vi "IO Module Testing.vi"() -> (0 "PIR":bool)   [LabVIEW 2015]
uses:
  <vilib>/rvi/interface/nirviOpenFPGA/nirviOpenFPGA.xnode
  <vilib>/rvi/interface/nirviMethod/nirviMethod.xnode
  <vilib>/FPGAPlugInAG/Dynamic/niLvFpga_Run_Dynamic.vi
  <vilib>/rvi/interface/nirviCloseFPGA/nirviCloseFPGA.xnode
  <vilib>/FPGAPlugInAG/Dynamic/niLvFpga_Close_Dynamic.vi
  FPGA Bitfiles/PDMSMain_FPGATarget-Wi-Fi_Express2_Jo8xc+hAvHc.lvbitx
  FPGA/Express.vi
  <vilib>/FPGAPlugInAG/myRIO-1900/niLvFpga_Open_myRIO-1900.vi
  <vilib>/rvi/interface/common/dynamic/niFpgaDynamicAddResources.vi
panel:
  out "Ultrasuond":cluster{"US BK":i16, "US FR":i16, "US FL":i16}
  out "Accelerometer":cluster{"Z":i16, "Y":i16, "X":i16}
  out "Button":bool
  out "Error Out":errorcluster
  in  "Error In":errorcluster
  in  "Stop Button":bool
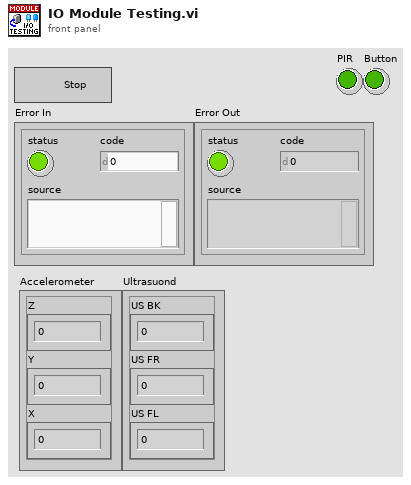
[diagram p1: front panel]
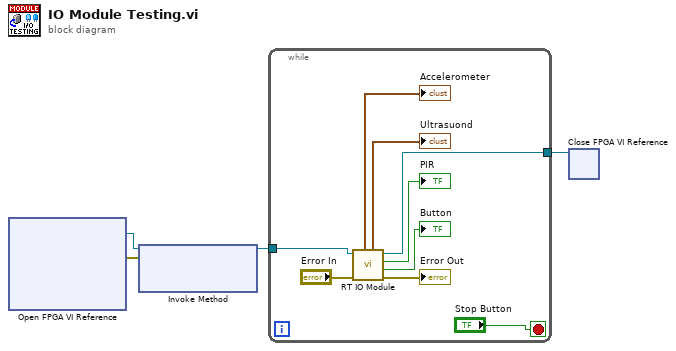
[diagram p0: block diagram]
diagram:
  n1 = xnode "Open FPGA VI Reference"() -> ("FPGA VI Reference Out"=w4:refnum<k20>, "error out"=w3:errorcluster)  [unwired: 2 in]
  n2 = xnode "Invoke Method"("FPGA VI Reference In"=w4, "error in"=w3) -> ("FPGA VI Reference Out"=w2:refnum<k20>)  [unwired: 1 in, 1 out]
  n3 = while {
    tunnel: w2 -> [w6]
    tunnel: [w5] -> w1
    stop <- "Stop Button" stop-if-true
    n4 = call "RT IO Module.vi"("Error In"="Error In", "FPGA VI Reference In"=w6) -> ("Error Out"=→"Error Out":errorcluster, "Button"=→"Button":bool, "PIR"=→"PIR":bool, "FPGA VI Reference Out"=w5:refnum<k20>, "Ultrasuond"=→"Ultrasuond":cluster{"US BK":i16, "US FR":i16, "US FL":i16}, "Accelerometer"=→"Accelerometer":cluster{"Z":i16, "Y":i16, "X":i16})  [unwired: 2 in]
  }
  n5 = xnode "Close FPGA VI Reference"("FPGA VI Reference In"=w1) -> ()  [unwired: 1 in, 1 out]
